vi "DrawPolarPlot.vi"(0 "reference in":refnum<class "LcWebView.lvclass">, 1 "XLabels":string[](array[string]), 2 "Polar.Dataset":dbl[][](array[numeric]), 3 "LinePlot.DatasetLabels":string[](array[string]), 5 "Error In":errorcluster, 6 "GenericPlotOptions":T1, 7 "BarPlot.PlotColours":u32[][](array[numeric])) -> (14 "reference out":refnum<class "LcWebView.lvclass">, 19 "Error Out":errorcluster)   [LabVIEW 2018, in "LcWebView.lvclass"]
uses:
  LcWebView.lvclass
  ctrls/GenericPlotOption.ctl
  ctrls/LegendPosition.ctl
  cdfa7b6c-348e-4618-b79e-b8b55caa0d01.vi
  <vilib>/JDP Science/JSONtext/Variant to JSON Text.vi
  <vilib>/JDP Science/JSONtext/LVClass Serializer/JSONtext LVClass Serializer.lvclass
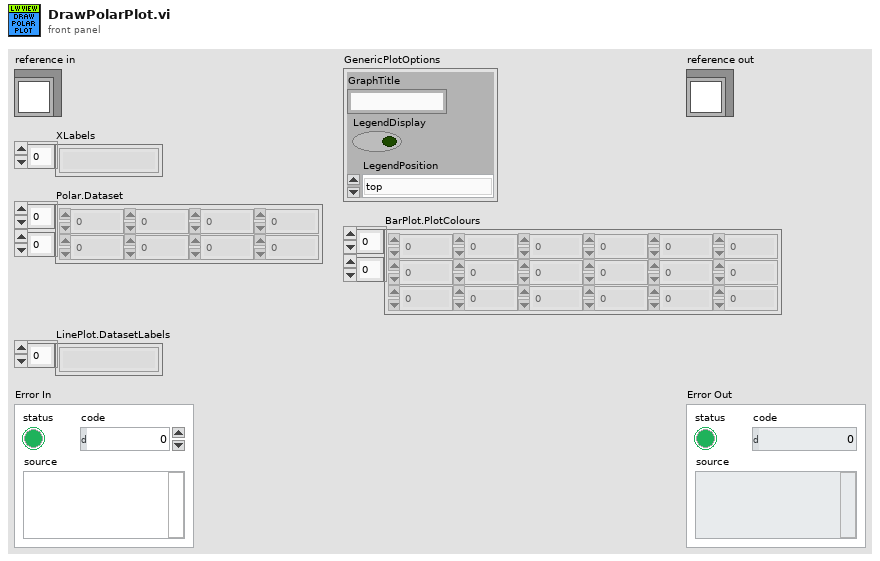
[diagram p1: front panel]
types:
  T1 = typedef "LcWebView.lvclass/GenericPlotOption.ctl" = cluster{"GraphTitle":string, "LegendDisplay":bool, "LegendPosition":T2}
  T2 = typedef "LcWebView.lvclass/LegendPosition.ctl" = enum16{"top", "right", "left", "bottom"}
  T3 = cluster{"action":string, "PlotData":string, "GenericPlotOptions":T1}
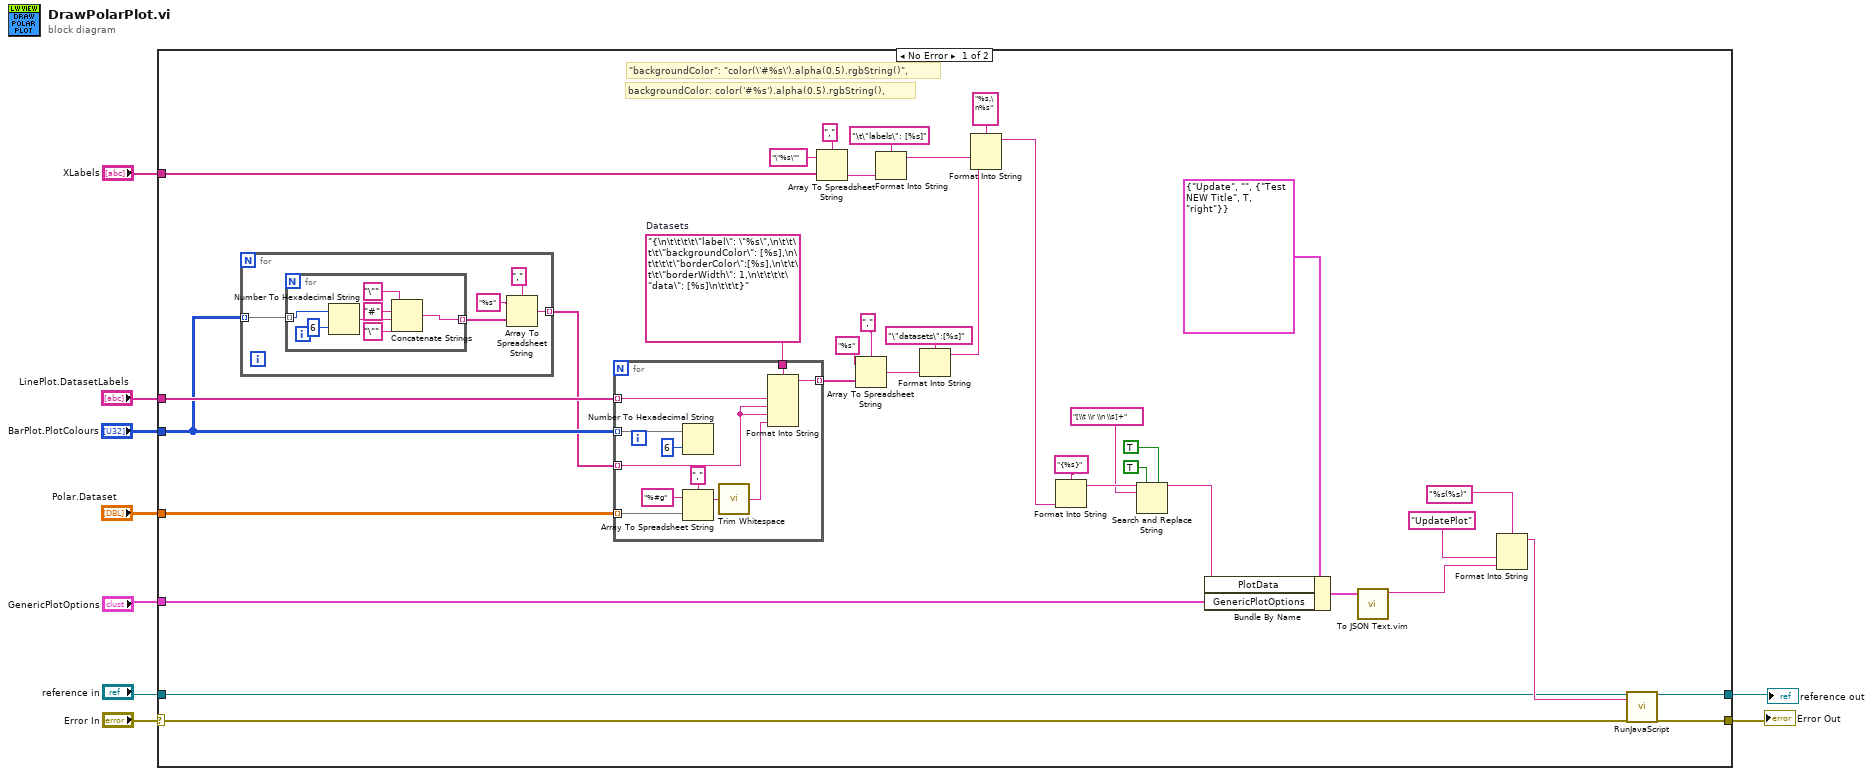
[diagram p0: block diagram]
diagram:
  n1 = case shown="No Error" "Error In" {
    selector: "Error In" -> [w16 w70]
    tunnel: [w17 w70] -> w1
    tunnel: [w18 w69] -> w2
    tunnel: "reference in" -> [w19 w69]
    tunnel: "Polar.Dataset" -> [w36 _]
    tunnel: "BarPlot.PlotColours" -> [w11 _]
    tunnel: "LinePlot.DatasetLabels" -> [w35 _]
    tunnel: "XLabels" -> [w34 _]
    tunnel: "GenericPlotOptions" -> [w26 _]
    frame No Error {
      w37 = "{\n\t\t\t\t\"label\": \"%s\",\n\t\t\t\t\"backgroundColor\": [%s],\n\t\t\t\t\"borderColor\":[%s],\n\t\t\t\t\"borderWidth\": 1,\n\t\t\t\t\"data\": [%s]\n\t\t\t}"  # Datasets
      # "\"backgroundColor\": \"color(\\'#%s\\').alpha(0.5).rgbString()\","
      # "backgroundColor: color('#%s').alpha(0.5).rgbString(),"
      n2 = for {
        tunnel: w11 -> [w50] mode=indexing
        tunnel: [w46] -> w10 mode=indexing
        n3 = for {
          tunnel: w50 -> [w56] mode=indexing
          tunnel: [w54] -> w47 mode=indexing
          n4 = Number To Hexadecimal String(1:i16 6 ("width (-)"), 2:w56) -> (0:w55:string)
          n5 = Concatenate Strings("\"" ("string"), "#" ("string"), w55, "\"" ("string")) -> (w54:string)
        }
        n6 = Array To Spreadsheet String(delimiter (Tab)="," ("separator"), array=w47, 3:"%s" ("format string")) -> (spreadsheet string=w46:string)
      }
      n7 = for {
        tunnel: w36 -> [w66] mode=indexing
        tunnel: w11 -> [w62] mode=indexing
        tunnel: w35 -> [w64] mode=indexing
        tunnel: [w63] -> w15 mode=indexing
        tunnel: w37 -> [w65]
        tunnel: w10 -> [w58] mode=indexing
        n8 = Number To Hexadecimal String(1:i16 6 ("width (-)"), 2:w62) -> ()  [unwired: 1 out]
        n9 = Array To Spreadsheet String(delimiter (Tab)=",", array=w66, 3:"%#g" ("format string")) -> (spreadsheet string=w61:string)
        n10 = call <vilib>:"Trim Whitespace.vi"("string"=w61) -> ("trimmed string"=w60:string)  [unwired: 1 in]
        n11 = Format Into String(format string=w65, w64, w58, w58, w60) -> (resulting string=w63:string)  [unwired: 2 in, 1 out]
      }
      n12 = Array To Spreadsheet String(delimiter (Tab)=",", array=w34, 3:"\"%s\"" ("format string")) -> (spreadsheet string=w41:string)
      n13 = Array To Spreadsheet String(delimiter (Tab)="," ("separator"), array=w15, 3:"%s" ("format string")) -> (spreadsheet string=w12:string)
      n14 = Format Into String(format string="\t\"labels\": [%s]", w41) -> (resulting string=w44:string)  [unwired: 2 in, 1 out]
      n15 = Format Into String(format string="\"datasets\":[%s]", w12) -> (resulting string=w39:string)  [unwired: 2 in, 1 out]
      n16 = Format Into String(format string="%s,\n%s", w44, w39) -> (resulting string=w32:string)  [unwired: 2 in, 1 out]
      n17 = Format Into String(format string="{%s}", w32) -> (resulting string=w31:string)  [unwired: 2 in, 1 out]
      n18 = Search and Replace String(replace all?=TRUE ("replace all? (F)"), multiline?=TRUE ("multiline? (F)"), input string=w31, search string="[\\t \\r \\n \\s]+") -> (result string=w30:string)  [unwired: 4 in, 3 out]
      n19 = Bundle By Name(cluster=T3 {"action"="Update", "PlotData"="", "GenericPlotOptions"={"GraphTitle"="Test NEW Title", "LegendDisplay"=TRUE, "LegendPosition"=enum."right"}}, "PlotData"=w30, "GenericPlotOptions"=w26) -> (w24:T3)
      n20 = call "To JSON Text.vim"("Anything"=w24) -> ("<JSON>"=w21:string)  [unwired: 9 in, 1 out]
      n21 = Format Into String(format string="%s(%s)", "UpdatePlot" ("input 1"), w21) -> (resulting string=w20:string)  [unwired: 2 in, 1 out]
      n22 = call-dynamic "RunJavaScript.vi"("reference in"=w19, "Java Script Function"=w20, "Error In"=w16) -> ("reference out"=w18:refnum<class "LcWebView.lvclass">, "Error Out"=w17:errorcluster)  [unwired: 13 in, 2 out]
    }
    frame Error {
    }
  }
  "Error Out" <- w1
  "reference out" <- w2
